vi "Step1PreviousY.vi"() -> ()   [LabVIEW 2025]
uses:
  <vilib>/Utility/file.llb/Read Delimited Spreadsheet (DBL).vi
  <vilib>/Analysis/NI_AALBase.lvlib
panel:
  out "After Outlier Removal":waveform(dbl)(graph)
  in  "Z Threshold":dbl
  in  "Data File Path":path
  out "Time vs Signal":waveform(dbl)(graph)
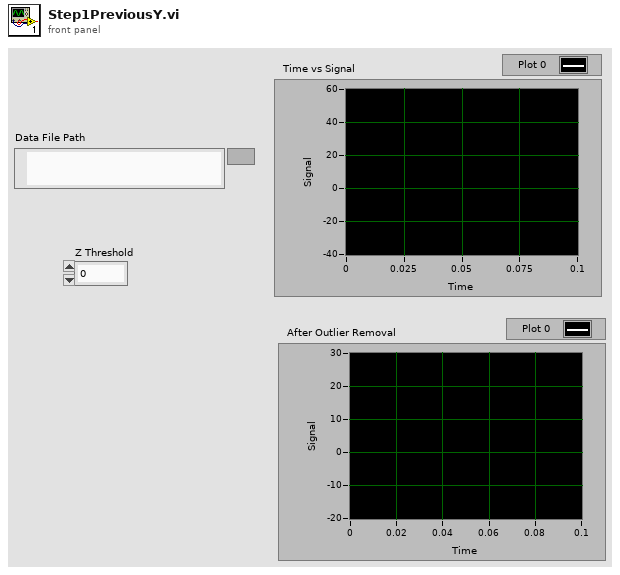
[diagram p1: front panel]
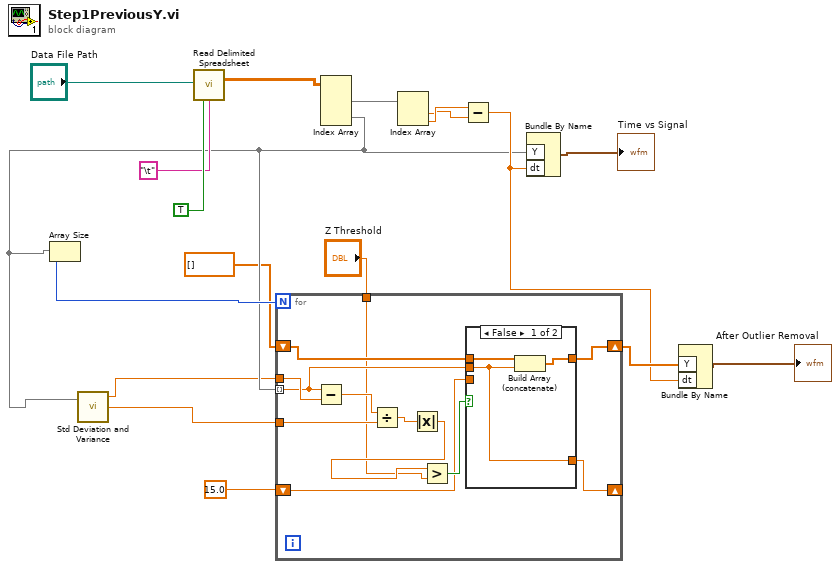
[diagram p0: block diagram]
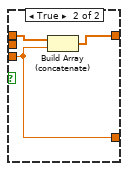
[diagram p2: hidden frame]
diagram:
  n1 = call-poly <vilib>:"Read Delimited Spreadsheet.vi"("file path (dialog if empty)"="Data File Path", "transpose? (F)"=TRUE, "delimiter (\\t)"="\t" ("delimiter (\\t)")) -> ("all rows"=w16:dbl[][])  [unwired: 7 in, 5 out]
  n2 = Index Array(array=w16) -> (element #1=w15:dbl[], element #2=w5:dbl[])  [unwired: 4 in]
  n3 = Array Size(array=w5) -> (size(s)=w6:i32)
  n4 = call <vilib>:"Std Deviation and Variance.vi"("X"=w5) -> ("mean"=w4:dbl, "standard deviation"=w3:dbl)  [unwired: 1 in, 1 out]
  n5 = for {
    N: w6 -> [_]
    shift-right: [w25] -> w9
    tunnel: w3 -> [w29]
    tunnel: w5 -> [w23] mode=indexing
    tunnel: w4 -> [w27]
    tunnel: "Z Threshold" -> [w19]
    shift-left: dbl[] [] -> [w24]
    shift-right: [w21] -> _
    shift-left: 15.0 -> [w22]
    n6 = Subtract(x=w23, y=w27) -> (x-y=w30:dbl)
    n7 = Divide(x=w30, y=w29) -> (x/y=w28:dbl)
    n8 = Absolute Value(x=w28) -> (abs(x)=w20:dbl)
    n9 = Greater?(x=w20, y=w19) -> (0:w26:bool)
    n10 = case shown="False" w26 {
      tunnel: w23 -> [w31 _]
      tunnel: w24 -> [w32 w36]
      tunnel: [w33 w35] -> w25
      tunnel: w22 -> [_ w34]
      tunnel: [w31 w34] -> w21
      frame False {
        n11 = Build Array (concatenate)(w32, w31) -> (w33:dbl[])
      }
      frame True {
        n12 = Build Array (concatenate)(w36, w34) -> (w35:dbl[])
      }
    }
  }
  n13 = Index Array(array=w15) -> (element #1=w13:dbl, element #2=w14:dbl)  [unwired: 2 in]
  n14 = Subtract(x=w14, y=w13) -> (x-y=w7:dbl)
  n15 = Bundle By Name("Y"=w5, "dt"=w7) -> (→"Time vs Signal":waveform(dbl))  [unwired: 1 in]
  n16 = Bundle By Name("Y"=w9, "dt"=w7) -> (→"After Outlier Removal":waveform(dbl))  [unwired: 1 in]
